vi "globalValue.vi"() -> ()   [LabVIEW 2019]
uses:
  03_Home/controller/pannelState.ctl
panel:
  out "*temp_userId":string
  out "robotSettingId":string
  out "patientsId":string
  out "traningId":string
  out "loginId":string
  out "userId":string
  out "roleId":string
  in  "State":T1
  in  "참조":refnum<vi>
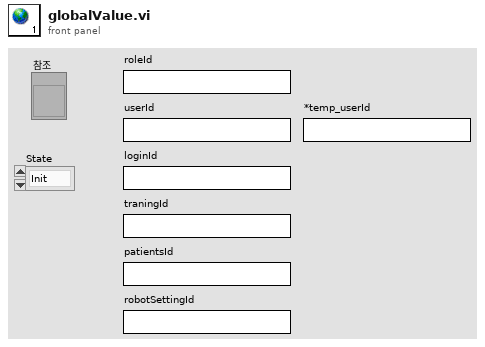
[diagram p1: front panel]
types:
  T1 = typedef "pannelState.ctl" = enum16{"Init", "LogIn", "SignUpView", "Home", "Management_patientList", "Management_patientTrashtList", "Management_patientCreate", "Management_patientUpdate", "Management_patientTraining", "Management_patientTrainingDetail", "H-MEDI PatientList", "H-MEDI HardwareCtl", "Adjust", "FineTuning", "UserList", "UserDetail", "Exit"}
diagram:
